vi "myRIO v1.0 Close AO.vi"(8 "error in (no error)":errorcluster, 9 "Scale Constants Array":T1, 10 "AO Channel List":T5, 11 "myRIO Ref In":T3) -> (0 "error out":errorcluster)   [LabVIEW 2021]
uses:
  <vilib>/myRIO/Common/Instrument Driver Framework/myRIO v1.0/AO/typedefs/AO Channels List.ctl
  <vilib>/myRIO/Common/Instrument Driver Framework/myRIO v1.0/AO/typedefs/AO Channels Enum.ctl
  <vilib>/myRIO/Common/Instrument Driver Framework/Utilities/typedefs/myRIO v1.0 Reference.ctl
  <vilib>/myRIO/Common/Instrument Driver Framework/Utilities/typedefs/Generic FPGA Reference.ctl
  <vilib>/myRIO/Common/Instrument Driver Framework/Utilities/typedefs/Analog Scaling Constants List.ctl
  <vilib>/myRIO/Common/Instrument Driver Framework/Utilities/typedefs/Analog Scaling Constants.ctl
  <vilib>/myRIO/Common/Instrument Driver Framework/myRIO v1.0/Resource Manager/vis/myRIO v1.0 Unreserve Channel List.vi
  <vilib>/myRIO/Common/Instrument Driver Framework/myRIO v1.0/AO/vis/myRIO v1.0 Build MUX Configuration AO.vi
  <vilib>/myRIO/Common/Instrument Driver Framework/myRIO v1.0/Resource Manager/vis/myRIO v1.0 Unreserve Channel.vi
  <vilib>/myRIO/Common/Instrument Driver Framework/myRIO v1.0/Resource Manager/vis/myRIO v1.0 Build Mutex Name.vi
  <vilib>/myRIO/Common/Instrument Driver Framework/Utilities/vis/Configuration Manager.vi
  <vilib>/myRIO/Common/Instrument Driver Framework/Utilities/vis/IO Manager.vi
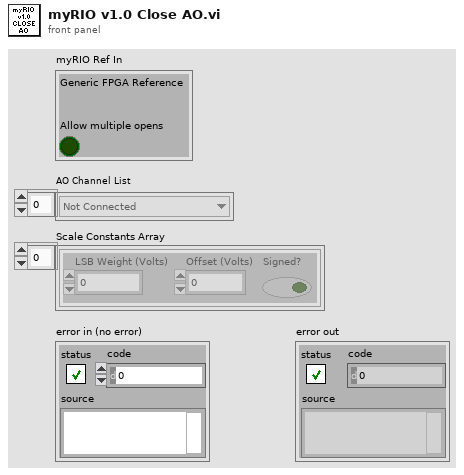
[diagram p1: front panel]
types:
  T1 = typedef "Analog Scaling Constants List.ctl" = T2[]
  T2 = typedef "Analog Scaling Constants.ctl" = cluster{"LSB Weight (Volts)":dbl, "Offset (Volts)":dbl, "Signed?":bool}
  T3 = typedef "myRIO v1.0 Reference.ctl" = cluster{"Generic FPGA Reference":T4, "Allow multiple opens":bool}
  T4 = typedef "Generic FPGA Reference.ctl" = refnum<k20>
  T5 = typedef "AO Channels List.ctl" = T6[]
  T6 = typedef "AO Channels Enum.ctl" = enum16{"Not Connected", "AudioOut/Left", "AudioOut/Right", "C/AO0", "C/AO1", "A/AO0", "A/AO1", "B/AO0", "B/AO1"}
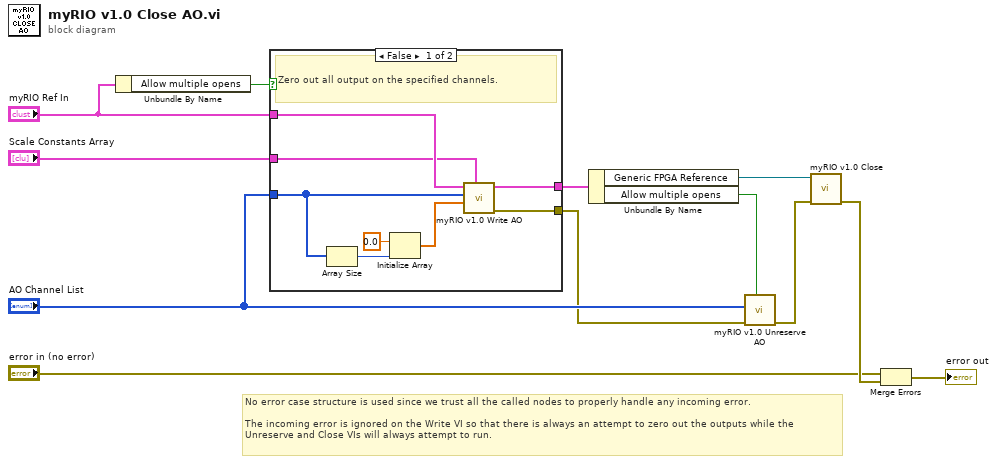
[diagram p0: block diagram]
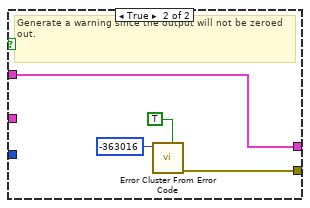
[diagram p2: hidden frame]
diagram:
  # "No error case structure is used since we trust all the called nodes to properly handle any incoming error.\n\nThe incoming error is ignored on the Write VI so that there is always an attempt to zero out the outputs while the Unreserve and Close VIs will always attempt to run."
  n1 = Unbundle By Name("myRIO Ref In") -> ("Allow multiple opens"=w4:bool)
  n2 = case shown="False" w4 {
    tunnel: "AO Channel List" -> [w18 _]
    tunnel: "myRIO Ref In" -> [w16 w23]
    tunnel: [w15 w23] -> w9
    tunnel: [w14 w24] -> w8
    tunnel: "Scale Constants Array" -> [w13 _]
    frame False {
      # "Zero out all output on the specified channels."
      n3 = Array Size(array=w18) -> (size(s)=w17:i32)
      n4 = Initialize Array(0.0 ("element"), w17) -> (w20:dbl[])
      n5 = call <vilib>:"myRIO v1.0 Write AO.vi"("Scale Constants Array"=w13, "dbl Scaled Value List"=w20, "Channel List"=w18, "myRIO Ref In"=w16) -> ("error out"=w14:errorcluster, "myRIO Ref Out"=w15:T3)  [unwired: 6 in]
    }
    frame True {
      # "Generate a warning since the output will not be zeroed out."
      n6 = call <vilib>:"Error Cluster From Error Code.vi"("is warning? (False)"=TRUE, "error code (0)"=-363016) -> ("error out"=w24:errorcluster)  [unwired: 7 in]
    }
  }
  n7 = Unbundle By Name(w9) -> ("Generic FPGA Reference"=w10:T4, "Allow multiple opens"=w3:bool)
  n8 = call <vilib>:"myRIO v1.0 Unreserve AO.vi"("Allow multiple opens?"=w3, "error in (no error)"=w8, "AI Channel List"="AO Channel List") -> ("error out"=w7:errorcluster)  [unwired: 8 in]
  n9 = call <vilib>:"myRIO v1.0 Close.vi"("error in (no error)"=w7, "myRIO FPGA Ref In"=w10) -> ("error out"=w6:errorcluster)  [unwired: 9 in]
  n10 = Merge Errors("error in (no error)", w6) -> (→"error out":errorcluster)
